vi "KGN Get Flow.vi"(8 "Fehler (Eingang, kein Fehler)":errorcluster, 9 "Info Cluster":T1, 10 "VISA-Referenz (Eingang)":refnum<visa-resource-name>, 11 "device (Eingang)":u32) -> (0 "Fehler (Ausgang)":errorcluster, 1 "Info Cluster out":T1, 2 "VISA-Referenz (Ausgang)":refnum<visa-resource-name>, 3 "dup device":u32, 4 "Flow Output Cluster (Ausgang)":T2, 6 "Kkommandos gesendet":string)   [LabVIEW 2020, in "Linearisierung v2.lvlib" / "Gasteiler.lvlib" / "HovaCAL_Interface.lvlib" / "KGN.lvlib" / "KGN GUI Get.lvlib"]
uses:
  KGN GUI Get.lvlib
  Controls/Info Cluster.ctl
  get/get.lvlib
  Controls/Controls.lvlib
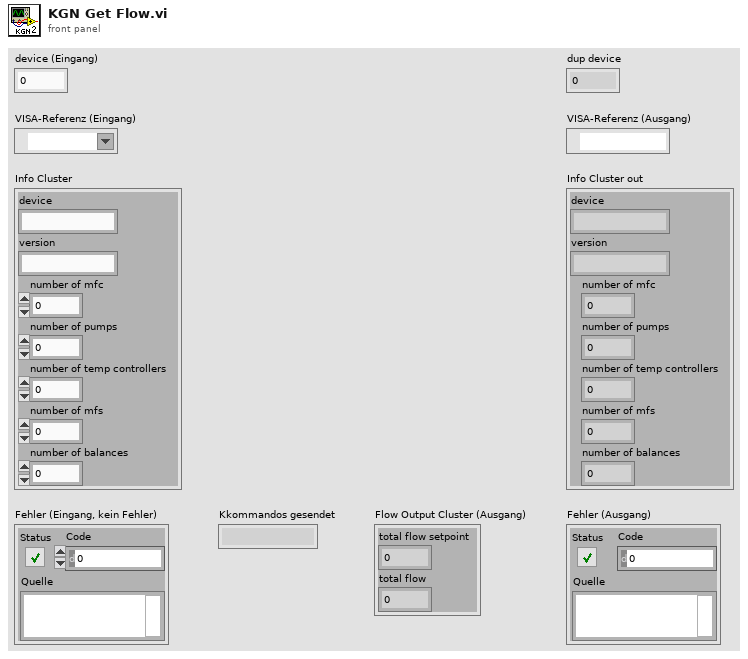
[diagram p1: front panel]
types:
  T1 = typedef "Linearisierung v2.lvlib/Gasteiler.lvlib/HovaCAL_Interface.lvlib/Controls.lvlib/Info Cluster.ctl" = cluster{"device":string, "version":string, "number of mfc":i32, "number of pumps":i32, "number of temp controllers":i32, "number of mfs":i32, "number of balances":i32}
  T2 = cluster{"total flow setpoint":dbl, "total flow":dbl}
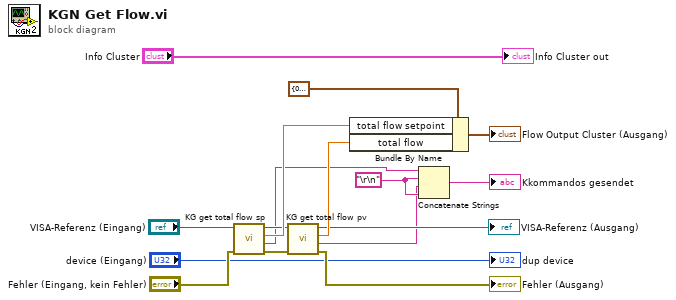
[diagram p0: block diagram]
diagram:
  w4 = "\r\n"
  n1 = call "KG get total flow sp.vi"("Fehler (Eingang, kein Fehler)"="Fehler (Eingang, kein Fehler)", "VISA-Ressourcenname"="VISA-Referenz (Eingang)") -> ("Fehler (Ausgang)"=w5:errorcluster, "Kommando gesendet"=w3:string, "total flow setpoint"=w15:dbl, "VISA-Ressourcenname (Ausgang)"=w6:refnum<visa-resource-name>)  [unwired: 6 in]
  n2 = call "KG get total flow pv.vi"("Fehler (Eingang, kein Fehler)"=w5, "VISA-Ressourcenname"=w6) -> ("Fehler (Ausgang)"=→"Fehler (Ausgang)":errorcluster, "Kommando gesendet"=w2:string, "total flow"=w12:dbl, "VISA-Ressourcenname (Ausgang)"=→"VISA-Referenz (Ausgang)":refnum<visa-resource-name>)  [unwired: 6 in]
  n3 = Bundle By Name(cluster=T2 {"total flow setpoint"=0.0, "total flow"=0.0} ("Flow Output Cluster (Ausgang)"), "total flow setpoint"=w15, "total flow"=w12) -> (→"Flow Output Cluster (Ausgang)":T2)
  n4 = Concatenate Strings(w3, w4, w2, w4) -> (→"Kkommandos gesendet":string)
  "dup device" <- "device (Eingang)"
  "Info Cluster out" <- "Info Cluster"
